vi "DHT12.vi"() -> ()   [LabVIEW 2020]
uses:
  <vilib>/MakerHub/LINX/Private/Device/Type Defs/TCP Config.ctl
  <vilib>/MakerHub/LINX/Private/Local IO/LinxI2cWrite.vi
  <vilib>/MakerHub/LINX/Public/Utilities/Check Channel.vi
  <vilib>/MakerHub/LINX/Public/Utilities/Open Serial.vi
  <vilib>/MakerHub/LINX/Public/Utilities/Open TCP.vi
  <vilib>/MakerHub/LINX/Private/Utilties/Generate Error.vi
  <vilib>/MakerHub/LINX/LMH-LINX.lvlib
  <vilib>/MakerHub/LINX/Private/Device/Device.lvlib
panel:
  out "Temperature":dbl
  in  "TCP Configuration":T1={"IP Address"="0.0.0.0", "Port"=44300}
  in  "Use TCP":bool
  in  "Serial Port":refnum<visa-resource-name>
  out "Loop Rate (Hz)":u32
  in  "Stop Button":bool
  out "Temperature Chart":dbl(graph)
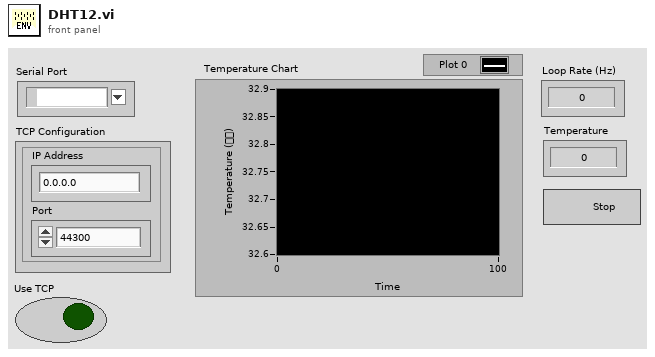
[diagram p1: front panel]
types:
  T1 = typedef "LMH-LINX.lvlib/Device.lvlib/TCP Config.ctl" = cluster{"IP Address":string, "Port":u16}
  T2 = typedef "LMH-LINX.lvlib/LINX Ref.ctl" = cluster{"IO":T3, "Interface":T4, "LINX Device Config":T5}
  T3 = typedef "LMH-LINX.lvlib/Platform.ctl" = enum16{"Remote", "Local"}
  T4 = typedef "LMH-LINX.lvlib/Interface.ctl" = enum16{"Serial", "TCP"}
  T5 = typedef "LMH-LINX.lvlib/Device.lvlib/LINX Device Config.ctl" = cluster{"Interface":T4, "COM Port":refnum<visa-resource-name>, "TCP Configuration":T1, "Device Family":u8, "Device ID":u8, "Device Name":string, "TCP Ref":refnum<k5>, "Channels":T6}
  T6 = typedef "LMH-LINX.lvlib/Channels.ctl" = cluster{"DI":u8[], "DO":u8[], "AI":u8[], "AO":u8[], "PWM":u8[], "QE":u8[], "UART":u8[], "I2C 2":u8[], "SPI":u8[], "CAN":u8[], "Servo":u8[], "AI Ref (V)":dbl, "AI Resolution (Bits)":u8, "AO Ref (V)":dbl, "AO Resolution (Bits)":u8}
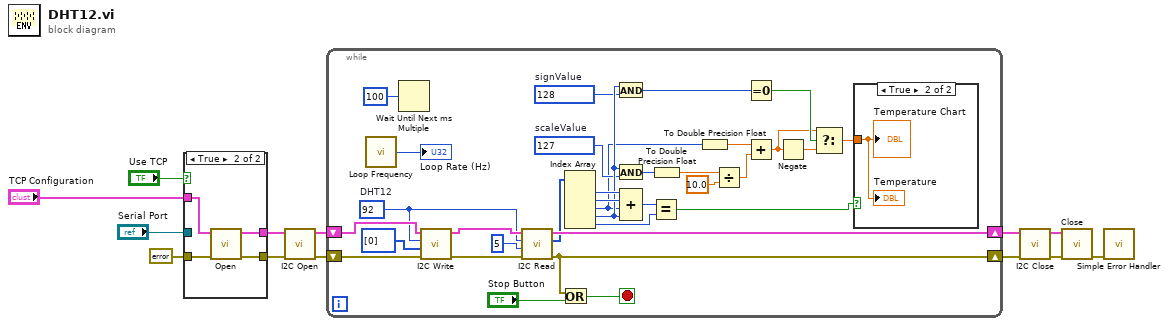
[diagram p0: block diagram]
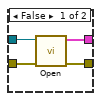
[diagram p2: hidden frame]
diagram:
  n1 = case shown="True" "Use TCP" {
    tunnel: [w15 w21] -> w2
    tunnel: [w16 w20] -> w1
    tunnel: errorcluster {"status"=FALSE, "code"=0, "source"=""} ("Error In") -> [w17 w19]
    tunnel: "Serial Port" -> [w14 _]
    tunnel: "TCP Configuration" -> [_ w18]
    frame False {
      n2 = call-poly <vilib>:"Open.vi"("Error In"=w17, "Serial Port"=w14) -> ("Error Out"=w16:errorcluster, "LINX Resource"=w15:T2)  [unwired: 7 in, 1 out]
    }
    frame True {
      n3 = call-poly <vilib>:"Open.vi"("Error In"=w19, "TCP Configuration"=w18) -> ("Error Out"=w20:errorcluster, "LINX Resource"=w21:T2)  [unwired: 7 in, 1 out]
    }
  }
  n4 = call <vilib>:"I2C Open.vi"("Error In"=w1, "LINX Resource"=w2) -> ("Error Out"=w11:errorcluster, "LINX Resource"=w12:T2)  [unwired: 8 in]
  n5 = while {
    shift-right: [w54] -> w10
    shift-left: w12 -> [w51]
    shift-right: [w26] -> w7
    shift-left: w11 -> [w50]
    stop <- w25 stop-if-true
    w39 = u8 128  # signValue
    w40 = u8 127  # scaleValue
    w47 = u8 92  # DHT12
    n6 = call <vilib>:"Loop Frequency.vi"() -> ("Loop Rate (Hz)"=→"Loop Rate (Hz)":u32)
    n7 = Wait Until Next ms Multiple(millisecond multiple=u32 100) -> ()  [unwired: 1 out]
    n8 = call <vilib>:"I2C Write.vi"("Error In"=w50, "Data"=u8[] [0], "I2C Slave Address (0)"=w47, "LINX Resource"=w51) -> ("Error Out"=w53:errorcluster, "LINX Resource"=w52:T2)  [unwired: 6 in]
    n9 = call <vilib>:"I2C Read.vi"("Error In"=w53, "Bytes To Read"=u8 5, "I2C Slave Address (0)"=w47, "LINX Resource"=w52) -> ("Error Out"=w26:errorcluster, "Data"=w46:u8[], "LINX Resource"=w54:T2)  [unwired: 5 in]
    n10 = Or(x=w26, y="Stop Button") -> (x .or. y?=w25:bool)
    n11 = Index Array(array=w46) -> (element #1=w45:u8, element #2=w44:u8, element #3=w33:u8, element #4=w41:u8, element #5=w42:u8)  [unwired: 5 in]
    n12 = And(x=w41, y=w39) -> (x .and. y?=w32:u8)
    n13 = And(x=w41, y=w40) -> (x .and. y?=w38:u8)
    n14 = Compound Arithmetic op=ADD(w45, w44, w33, w41) -> (w43:u8)
    n15 = Equal?(x=w43, y=w42) -> (x = y?=w22:bool)
    n16 = To Double Precision Float(number=w38) -> (double precision float=w37:dbl)
    n17 = To Double Precision Float(number=w33) -> (double precision float=w34:dbl)
    n18 = Divide(x=w37, y=10.0) -> (x/y=w35:dbl)
    n19 = Equal To 0?(x=w32) -> (x = 0?=w31:bool)
    n20 = Add(x=w34, y=w35) -> (x+y=w29:dbl)
    n21 = Negate(x=w29) -> (-x=w30:dbl)
    n22 = Select(t=w29, s=w31, f=w30) -> (s? t:f=w24:dbl)
    n23 = case shown="True" w22 {
      tunnel: w24 -> [_ w55]
      frame False {
      }
      frame True {
        "Temperature Chart" <- w55
        "Temperature" <- w55
      }
    }
  }
  n24 = call <vilib>:"I2C Close.vi"("Error In"=w7, "LINX Resource"=w10) -> ("Error Out"=w8:errorcluster, "LINX Resource"=w9:T2)  [unwired: 8 in]
  n25 = call <vilib>:"Close.vi"("Error In"=w8, "LINX Resource"=w9) -> ("Error Out"=w13:errorcluster)  [unwired: 9 in]
  n26 = call <vilib>:"Simple Error Handler.vi"("error in (no error)"=w13) -> ()  [unwired: 4 in, 5 out]
